vi "1.vi"   [LabVIEW 2020]
panel:
  # "1"
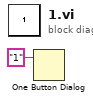
[diagram p0: block diagram]
diagram:
  n1 = One Button Dialog(message="1") -> ()  [unwired: 1 in, 1 out]
